vi "Arduino_susensoru.vi"() -> ()   [LabVIEW 2018]
uses:
  <vilib>/LabVIEW Interface for Arduino/Type Defs/Board Type.ctl
  <vilib>/LabVIEW Interface for Arduino/Type Defs/Connection Type.ctl
  <vilib>/LabVIEW Interface for Arduino/LabVIEW Interface for Arduino.lvlib
panel:
  out "Dolu":bool
  out "Nemli":bool
  out "Kuru":bool
  out "Nem ölçümü":dbl(slide) scale=0.0..100.0
  out "Numeric":i32
  in  "Analog Input Pin (0)":u8
  in  "stop":bool
  # "Hamid shah 170519921"
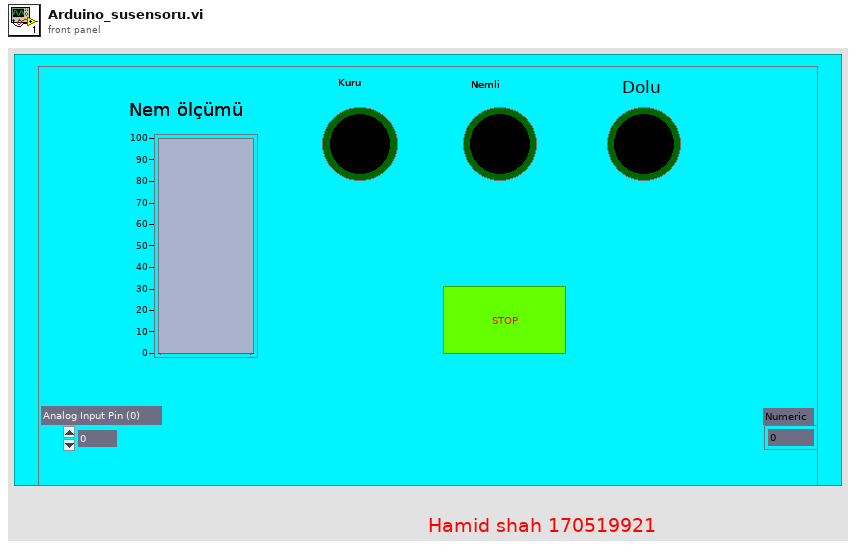
[diagram p1: front panel]
types:
  T1 = typedef "LabVIEW Interface for Arduino.lvlib/Connection Type.ctl" = enum8{"USB / Serial", "XBEE", "BlueSmirf (Bluetooth)"}
  T2 = typedef "LabVIEW Interface for Arduino.lvlib/Board Type.ctl" = enum16{"Uno", "Mega 2560"}
  T3 = typedef "LabVIEW Interface for Arduino.lvlib/Arduino Resource.ctl" = cluster{"VISA resource":refnum<visa-resource-name>, "Board Type":T2, "Connection Type":enum8{"USB / Serial"}, "Bytes Per Packet (15)":u8}
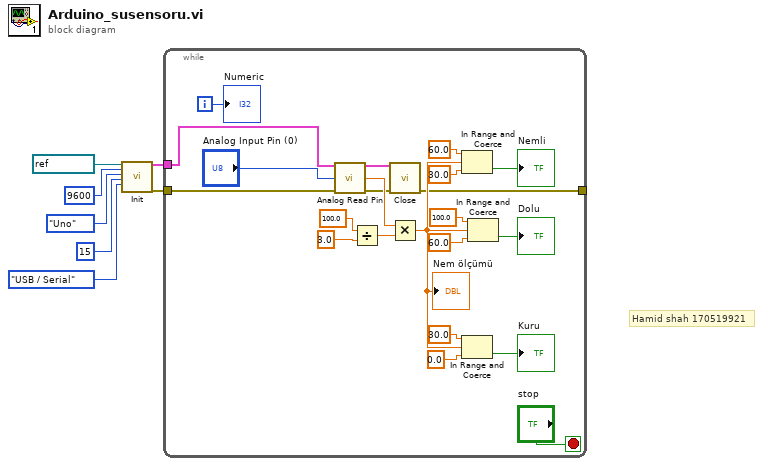
[diagram p0: block diagram]
diagram:
  # "Hamid shah 170519921"
  n1 = call <vilib>:"Init.vi"("VISA resource"=refnum<visa-resource-name> "COM7", "Baud Rate (115200)"=u32 9600, "Board Type (Uno)"=Board_Type."Uno", "Bytes Per Packet (15)"=u32 15, "Connection Type (USB/Serial)"=Connection_Type."USB / Serial") -> ("Arduino Resource"=w2:T3, "error out"=w1:errorcluster)  [unwired: 13 in]
  n2 = while {
    tunnel: w2 -> [w26]
    tunnel: w1 -> [w25]
    tunnel: [w11] -> _
    i -> [w27]
    stop <- "stop" stop-if-true
    n3 = call <vilib>:"Analog Read Pin.vi"("Arduino Resource"=w26, "Analog Input Pin (0)"="Analog Input Pin (0)", "error in"=w25) -> ("Arduino Resource"=w9:T3, "Voltage"=w24:dbl, "error out"=w8:errorcluster)  [unwired: 10 in]
    n4 = Divide(x=100.0, y=3.0) -> (x/y=w21:dbl)
    n5 = call <vilib>:"Close.vi"("Arduino Resource"=w9, "error in"=w8) -> ("error out"=w11:errorcluster)  [unwired: 13 in]
    n6 = Multiply(x=w24, y=w21) -> (x*y=w20:dbl)
    "Nem ölçümü" <- w20
    n7 = In Range and Coerce(upper limit=60.0, x=w20, lower limit=30.0) -> (In Range?=→"Nemli":bool)  [unwired: 1 out]
    n8 = In Range and Coerce(upper limit=30.0, x=w20, lower limit=0.0) -> (In Range?=→"Kuru":bool)  [unwired: 1 out]
    n9 = In Range and Coerce(upper limit=100.0, x=w20, lower limit=60.0) -> (In Range?=→"Dolu":bool)  [unwired: 1 out]
    "Numeric" <- w27
  }
